vi "ArraySubstraction.vi"(10 "Y [in]":dbl[](array[numeric]), 11 "X [in]":dbl[](array[numeric])) -> (3 "Array[out]":dbl[](array[numeric]))   [LabVIEW 2013]
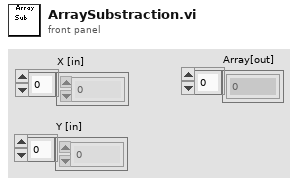
[diagram p1: front panel]
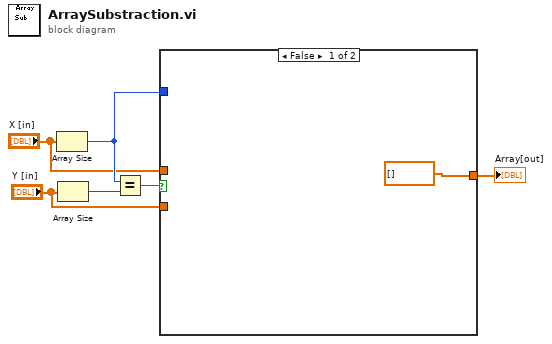
[diagram p0: block diagram]
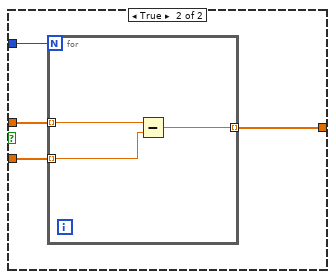
[diagram p2: hidden frame]
diagram:
  n1 = Array Size(array="X [in]") -> (size(s)=w3:i32)
  n2 = Array Size(array="Y [in]") -> (size(s)=w4:i32)
  n3 = Equal?(x=w3, y=w4) -> (x = y?=w5:bool)
  n4 = case shown="False" w5 {
    tunnel: [dbl[] [] ("Array[out]") w8] -> w6
    tunnel: w3 -> [_ w11]
    tunnel: "X [in]" -> [_ w10]
    tunnel: "Y [in]" -> [_ w9]
    frame False {
    }
    frame True {
      n5 = for {
        N: w11 -> [_]
        tunnel: w10 -> [w14] mode=indexing
        tunnel: w9 -> [w13] mode=indexing
        tunnel: [w12] -> w8 mode=indexing
        n6 = Subtract(x=w14, y=w13) -> (x-y=w12:dbl)
      }
    }
  }
  "Array[out]" <- w6
